vi "4.1 CSM API String to Numeric - Floating.vi"() -> ()   [LabVIEW 2017]
uses:
  63d4ee60-3d36-44f6-9846-d3c89712fa4e.vi
  5d5e870e-b8ec-4111-8fcd-715cbb1e366c.vi
  6ca2ea0b-5a64-4cad-9736-18ec21bbeae0.vi
  4ee676fc-47c0-4be0-9ff8-88677d132e6f.vi
  a152669e-7808-472e-ac68-82058263c032.vi
  API-String-Arugments-Support/_Support/Data To API String Arguments.vi
  API-String-Arugments-Support/_Support/Convert API String Arguments to Data(variant).vi
panel:
  out "Array 3":T1(array[cluster])=[{"Inplut String (Arguments)"="1", "Data"=1.0, "error"={"status"=FALSE, "code"=0, "source"=""}}, {"Inplut String (Arguments)"="10", "Data"=10.0, "error"={"status"=FALSE, "code"=0, "source"=""}}, {"Inplut String (Arguments)"="100", "Data"=100.0, "error"={"status"=FALSE, "code"=0, "source"=""}}, {"Inplut String (Arguments)"="1000", "Data"=1000.0, "error"={"status"=FALSE, "code"=0, "source"=""}}, {"Inplut String (Arguments)"="10000", "Data"=10000.0, "error"={"status"=FALSE, "code"=0, "source"=""}}, {"Inplut String (Arguments)"="100000", "Data"=100000.0, "error"={"status"=FALSE, "code"=0, "source"=""}}, {"Inplut String (Arguments)"="1000000", "Data"=1000000.0, "error"={"status"=FALSE, "code"=0, "source"=""}}, {"Inplut String (Arguments)"="10000000", "Data"=10000000.0, "error"={"status"=FALSE, "code"=0, "source"=""}}, {"Inplut String (Arguments)"="100000000", "Data"=100000000.0, "error"={"status"=FALSE, "code"=0, "source"=""}}, {"Inplut String (Arguments)"="1000000000", "Data"=1000000000.0, "error"={"status"=FALSE, "code"=0, "source"=""}}, {"Inplut String (Arguments)"="10000000000", "Data"=10000000000.0, "error"={"status"=FALSE, "code"=0, "source"=""}}, {"Inplut String (Arguments)"="100000000000", "Data"=100000000000.0, "error"={"status"=FALSE, "code"=0, "source"=""}}, {"Inplut String (Arguments)"="1000000000000", "Data"=1000000000000.0, "error"={"status"=FALSE, "code"=0, "source"=""}}, {"Inplut String (Arguments)"="10000000000000", "Data"=10000000000000.0, "error"={"status"=FALSE, "code"=0, "source"=""}}, {"Inplut String (Arguments)"="100000000000000", "Data"=100000000000000.0, "error"={"status"=FALSE, "code"=0, "source"=""}}, {"Inplut String (Arguments)"="1000000000000000", "Data"=1000000000000000.0, "error"={"status"=FALSE, "code"=0, "source"=""}}, {"Inplut String (Arguments)"="10000000000000000", "Data"=1e+16, "error"={"status"=FALSE, "code"=0, "source"=""}}, {"Inplut String (Arguments)"="100000000000000000", "Data"=1e+17, "error"={"status"=FALSE, "code"=0, "source"=""}}, {"Inplut String (Arguments)"="1000000000000000000", "Data"=1e+18, "error"={"status"=FALSE, "code"=0, "source"=""}}, {"Inplut String (Arguments)"="10000000000000000000", "Data"=1e+19, "error"={"status"=FALSE, "code"=0, "source"=""}}, {"Inplut String (Arguments)"="100000000000000000000", "Data"=1e+20, "error"={"status"=FALSE, "code"=0, "source"=""}}, {"Inplut String (Arguments)"="1000000000000000000000", "Data"=1e+21, "error"={"status"=FALSE, "code"=0, "source"=""}}, {"Inplut String (Arguments)"="10000000000000000000000", "Data"=1e+22, "error"={"status"=FALSE, "code"=0, "source"=""}}, {"Inplut String (Arguments)"="100000000000000000000000", "Data"=1e+23, "error"={"status"=FALSE, "code"=0, "source"=""}}, {"Inplut String (Arguments)"="1000000000000000000000000", "Data"=1e+24, "error"={"status"=FALSE, "code"=0, "source"=""}}, {"Inplut String (Arguments)"="10000000000000000000000000", "Data"=1e+25, "error"={"status"=FALSE, "code"=0, "source"=""}}, {"Inplut String (Arguments)"="100000000000000000000000000", "Data"=1e+26, "error"={"status"=FALSE, "code"=0, "source"=""}}, {"Inplut String (Arguments)"="1000000000000000000000000000", "Data"=1e+27, "error"={"status"=FALSE, "code"=0, "source"=""}}, {"Inplut String (Arguments)"="10000000000000000000000000000", "Data"=1e+28, "error"={"status"=FALSE, "code"=0, "source"=""}}, {"Inplut String (Arguments)"="100000000000000000000000000000", "Data"=1e+29, "error"={"status"=FALSE, "code"=0, "source"=""}}, {"Inplut String (Arguments)"="1000000000000000000000000000000", "Data"=1e+30, "error"={"status"=FALSE, "code"=0, "source"=""}}, {"Inplut String (Arguments)"="10000000000000000000000000000000", "Data"=1e+31, "error"={"status"=FALSE, "code"=0, "source"=""}}, {"Inplut String (Arguments)"="100000000000000000000000000000000", "Data"=1e+32, "error"={"status"=FALSE, "code"=0, "source"=""}}, {"Inplut String (Arguments)"="1000000000000000000000000000000000", "Data"=1e+33, "error"={"status"=FALSE, "code"=0, "source"=""}}, {"Inplut String (Arguments)"="10000000000000000000000000000000000", "Data"=1e+34, "error"={"status"=FALSE, "code"=0, "source"=""}}] {"Data" format="%#_6e"}
  out "Multiplication Display":T2(array[cluster])=[{"Float Value"=10.001, "Flatten String"="10.001", "Retrieve Float"=10.001, "error"={"status"=FALSE, "code"=0, "source"=""}}, {"Float Value"=100.00999999999999, "Flatten String"="100.01", "Retrieve Float"=100.01, "error"={"status"=FALSE, "code"=0, "source"=""}}, {"Float Value"=1000.0999999999999, "Flatten String"="1.0001k", "Retrieve Float"=1000.1, "error"={"status"=FALSE, "code"=0, "source"=""}}, {"Float Value"=10001.0, "Flatten String"="10.001k", "Retrieve Float"=10001.0, "error"={"status"=FALSE, "code"=0, "source"=""}}, {"Float Value"=100010.0, "Flatten String"="100.01k", "Retrieve Float"=100010.0, "error"={"status"=FALSE, "code"=0, "source"=""}}, {"Float Value"=1000100.0, "Flatten String"="1.0001M", "Retrieve Float"=1000100.0, "error"={"status"=FALSE, "code"=0, "source"=""}}, {"Float Value"=10001000.0, "Flatten String"="10.001M", "Retrieve Float"=10001000.0, "error"={"status"=FALSE, "code"=0, "source"=""}}, {"Float Value"=100010000.0, "Flatten String"="100.01M", "Retrieve Float"=100010000.0, "error"={"status"=FALSE, "code"=0, "source"=""}}, {"Float Value"=1000100000.0, "Flatten String"="1.0001G", "Retrieve Float"=1000100000.0, "error"={"status"=FALSE, "code"=0, "source"=""}}, {"Float Value"=10001000000.0, "Flatten String"="10.001G", "Retrieve Float"=10001000000.0, "error"={"status"=FALSE, "code"=0, "source"=""}}, {"Float Value"=100010000000.0, "Flatten String"="100.01G", "Retrieve Float"=100010000000.0, "error"={"status"=FALSE, "code"=0, "source"=""}}, {"Float Value"=1000100000000.0, "Flatten String"="1.0001T", "Retrieve Float"=1000100000000.0, "error"={"status"=FALSE, "code"=0, "source"=""}}, {"Float Value"=10001000000000.0, "Flatten String"="10.001T", "Retrieve Float"=10001000000000.0, "error"={"status"=FALSE, "code"=0, "source"=""}}, {"Float Value"=100010000000000.0, "Flatten String"="100.01T", "Retrieve Float"=100010000000000.0, "error"={"status"=FALSE, "code"=0, "source"=""}}, {"Float Value"=1000100000000000.0, "Flatten String"="1.0001P", "Retrieve Float"=1000100000000000.0, "error"={"status"=FALSE, "code"=0, "source"=""}}, {"Float Value"=1.0001e+16, "Flatten String"="10.001P", "Retrieve Float"=1.0001e+16, "error"={"status"=FALSE, "code"=0, "source"=""}}, {"Float Value"=1.0001e+17, "Flatten String"="100.01P", "Retrieve Float"=1.0001e+17, "error"={"status"=FALSE, "code"=0, "source"=""}}, {"Float Value"=1.0001e+18, "Flatten String"="1.0001E", "Retrieve Float"=1.0001e+18, "error"={"status"=FALSE, "code"=0, "source"=""}}, {"Float Value"=1.0001e+19, "Flatten String"="10.001E", "Retrieve Float"=1.0001e+19, "error"={"status"=FALSE, "code"=0, "source"=""}}, {"Float Value"=1.0001e+20, "Flatten String"="100.01E", "Retrieve Float"=1.0001e+20, "error"={"status"=FALSE, "code"=0, "source"=""}}, {"Float Value"=1.0001e+21, "Flatten String"="1.0001Z", "Retrieve Float"=1.0001e+21, "error"={"status"=FALSE, "code"=0, "source"=""}}, {"Float Value"=1.0001e+22, "Flatten String"="10.001Z", "Retrieve Float"=1.0001e+22, "error"={"status"=FALSE, "code"=0, "source"=""}}, {"Float Value"=1.0001e+23, "Flatten String"="100.01Z", "Retrieve Float"=1.0001000000000001e+23, "error"={"status"=FALSE, "code"=0, "source"=""}}, {"Float Value"=1.0000999999999999e+24, "Flatten String"="1.0001Y", "Retrieve Float"=1.0000999999999999e+24, "error"={"status"=FALSE, "code"=0, "source"=""}}, {"Float Value"=1.0001e+25, "Flatten String"="10.001Y", "Retrieve Float"=1.0001e+25, "error"={"status"=FALSE, "code"=0, "source"=""}}, {"Float Value"=1.0001e+26, "Flatten String"="100.01Y", "Retrieve Float"=1.0001000000000001e+26, "error"={"status"=FALSE, "code"=0, "source"=""}}, {"Float Value"=1.0001e+27, "Flatten String"="1.000100E+27", "Retrieve Float"=1.0001e+27, "error"={"status"=FALSE, "code"=0, "source"=""}}, {"Float Value"=1.0001e+28, "Flatten String"="10.001000E+27", "Retrieve Float"=1.0000999999999999e+28, "error"={"status"=FALSE, "code"=0, "source"=""}}, {"Float Value"=1.0001e+29, "Flatten String"="100.010000E+27", "Retrieve Float"=1.0001e+29, "error"={"status"=FALSE, "code"=0, "source"=""}}, {"Float Value"=1.0001e+30, "Flatten String"="1.000100E+30", "Retrieve Float"=1.0001e+30, "error"={"status"=FALSE, "code"=0, "source"=""}}, {"Float Value"=1.0001e+31, "Flatten String"="10.001000E+30", "Retrieve Float"=1.0001e+31, "error"={"status"=FALSE, "code"=0, "source"=""}}, {"Float Value"=1.0001e+32, "Flatten String"="100.010000E+30", "Retrieve Float"=1.0001000000000001e+32, "error"={"status"=FALSE, "code"=0, "source"=""}}, {"Float Value"=1.0001e+33, "Flatten String"="1.000100E+33", "Retrieve Float"=1.0001e+33, "error"={"status"=FALSE, "code"=0, "source"=""}}, {"Float Value"=1.0001e+34, "Flatten String"="10.001000E+33", "Retrieve Float"=1.0000999999999999e+34, "error"={"status"=FALSE, "code"=0, "source"=""}}, {"Float Value"=1.0001e+35, "Flatten String"="100.010000E+33", "Retrieve Float"=1.0001e+35, "error"={"status"=FALSE, "code"=0, "source"=""}}] {"Float Value" format="%#_6e"; "Retrieve Float" format="%#_6e"}
  out "Division Demonstration":T2(array[cluster])=[{"Float Value"=0.10001, "Flatten String"="100.01m", "Retrieve Float"=0.10001, "error"={"status"=FALSE, "code"=0, "source"=""}}, {"Float Value"=0.010001, "Flatten String"="10.001m", "Retrieve Float"=0.010001, "error"={"status"=FALSE, "code"=0, "source"=""}}, {"Float Value"=0.0010000999999999999, "Flatten String"="1.0001m", "Retrieve Float"=0.0010001, "error"={"status"=FALSE, "code"=0, "source"=""}}, {"Float Value"=0.00010000999999999999, "Flatten String"="100.01u", "Retrieve Float"=0.00010001, "error"={"status"=FALSE, "code"=0, "source"=""}}, {"Float Value"=1.0000999999999998e-05, "Flatten String"="10.001u", "Retrieve Float"=1.0001e-05, "error"={"status"=FALSE, "code"=0, "source"=""}}, {"Float Value"=1.0000999999999998e-06, "Flatten String"="1.0001u", "Retrieve Float"=1.0001e-06, "error"={"status"=FALSE, "code"=0, "source"=""}}, {"Float Value"=1.0000999999999998e-07, "Flatten String"="100.01n", "Retrieve Float"=1.0001000000000001e-07, "error"={"status"=FALSE, "code"=0, "source"=""}}, {"Float Value"=1.0000999999999998e-08, "Flatten String"="10.001n", "Retrieve Float"=1.0001e-08, "error"={"status"=FALSE, "code"=0, "source"=""}}, {"Float Value"=1.0000999999999999e-09, "Flatten String"="1.0001n", "Retrieve Float"=1.0001e-09, "error"={"status"=FALSE, "code"=0, "source"=""}}, {"Float Value"=1.0000999999999999e-10, "Flatten String"="100.01p", "Retrieve Float"=1.0001e-10, "error"={"status"=FALSE, "code"=0, "source"=""}}, {"Float Value"=1.0000999999999998e-11, "Flatten String"="10.001p", "Retrieve Float"=1.0001e-11, "error"={"status"=FALSE, "code"=0, "source"=""}}, {"Float Value"=1.0000999999999997e-12, "Flatten String"="1.0001p", "Retrieve Float"=1.0001e-12, "error"={"status"=FALSE, "code"=0, "source"=""}}, {"Float Value"=1.0000999999999997e-13, "Flatten String"="100.01f", "Retrieve Float"=1.0001000000000001e-13, "error"={"status"=FALSE, "code"=0, "source"=""}}, {"Float Value"=1.0000999999999997e-14, "Flatten String"="10.001f", "Retrieve Float"=1.0001e-14, "error"={"status"=FALSE, "code"=0, "source"=""}}, {"Float Value"=1.0000999999999996e-15, "Flatten String"="1.0001f", "Retrieve Float"=1.0001e-15, "error"={"status"=FALSE, "code"=0, "source"=""}}, {"Float Value"=1.0000999999999996e-16, "Flatten String"="100.01a", "Retrieve Float"=1.0001000000000001e-16, "error"={"status"=FALSE, "code"=0, "source"=""}}, {"Float Value"=1.0000999999999996e-17, "Flatten String"="10.001a", "Retrieve Float"=1.0001e-17, "error"={"status"=FALSE, "code"=0, "source"=""}}, {"Float Value"=1.0000999999999996e-18, "Flatten String"="1.0001a", "Retrieve Float"=1.0001e-18, "error"={"status"=FALSE, "code"=0, "source"=""}}, {"Float Value"=1.0000999999999995e-19, "Flatten String"="100.01z", "Retrieve Float"=1.0000999999999999e-19, "error"={"status"=FALSE, "code"=0, "source"=""}}, {"Float Value"=1.0000999999999996e-20, "Flatten String"="10.001z", "Retrieve Float"=1.0000999999999999e-20, "error"={"status"=FALSE, "code"=0, "source"=""}}, {"Float Value"=1.0000999999999995e-21, "Flatten String"="1.0001z", "Retrieve Float"=1.0001e-21, "error"={"status"=FALSE, "code"=0, "source"=""}}, {"Float Value"=1.0000999999999995e-22, "Flatten String"="100.01y", "Retrieve Float"=1.0001e-22, "error"={"status"=FALSE, "code"=0, "source"=""}}, {"Float Value"=1.0000999999999995e-23, "Flatten String"="10.001y", "Retrieve Float"=1.0000999999999998e-23, "error"={"status"=FALSE, "code"=0, "source"=""}}, {"Float Value"=1.0000999999999995e-24, "Flatten String"="1.0001y", "Retrieve Float"=1.0000999999999998e-24, "error"={"status"=FALSE, "code"=0, "source"=""}}, {"Float Value"=1.0000999999999995e-25, "Flatten String"="100.010000E-27", "Retrieve Float"=1.0001000000000001e-25, "error"={"status"=FALSE, "code"=0, "source"=""}}, {"Float Value"=1.0000999999999995e-26, "Flatten String"="10.001000E-27", "Retrieve Float"=1.0001e-26, "error"={"status"=FALSE, "code"=0, "source"=""}}, {"Float Value"=1.0000999999999995e-27, "Flatten String"="1.000100E-27", "Retrieve Float"=1.0001e-27, "error"={"status"=FALSE, "code"=0, "source"=""}}, {"Float Value"=1.0000999999999995e-28, "Flatten String"="100.010000E-30", "Retrieve Float"=1.0001000000000002e-28, "error"={"status"=FALSE, "code"=0, "source"=""}}, {"Float Value"=1.0000999999999995e-29, "Flatten String"="10.001000E-30", "Retrieve Float"=1.0001000000000001e-29, "error"={"status"=FALSE, "code"=0, "source"=""}}, {"Float Value"=1.0000999999999995e-30, "Flatten String"="1.000100E-30", "Retrieve Float"=1.0001e-30, "error"={"status"=FALSE, "code"=0, "source"=""}}, {"Float Value"=1.0000999999999994e-31, "Flatten String"="100.010000E-33", "Retrieve Float"=1.0001e-31, "error"={"status"=FALSE, "code"=0, "source"=""}}, {"Float Value"=1.0000999999999994e-32, "Flatten String"="10.001000E-33", "Retrieve Float"=1.0001e-32, "error"={"status"=FALSE, "code"=0, "source"=""}}, {"Float Value"=1.0000999999999995e-33, "Flatten String"="1.000100E-33", "Retrieve Float"=1.0001e-33, "error"={"status"=FALSE, "code"=0, "source"=""}}, {"Float Value"=1.0000999999999995e-34, "Flatten String"="100.010000E-36", "Retrieve Float"=1.0001e-34, "error"={"status"=FALSE, "code"=0, "source"=""}}, {"Float Value"=1.0000999999999996e-35, "Flatten String"="10.001000E-36", "Retrieve Float"=1.0001e-35, "error"={"status"=FALSE, "code"=0, "source"=""}}] {"Float Value" format="%#_6e"; "Retrieve Float" format="%#_6e"}
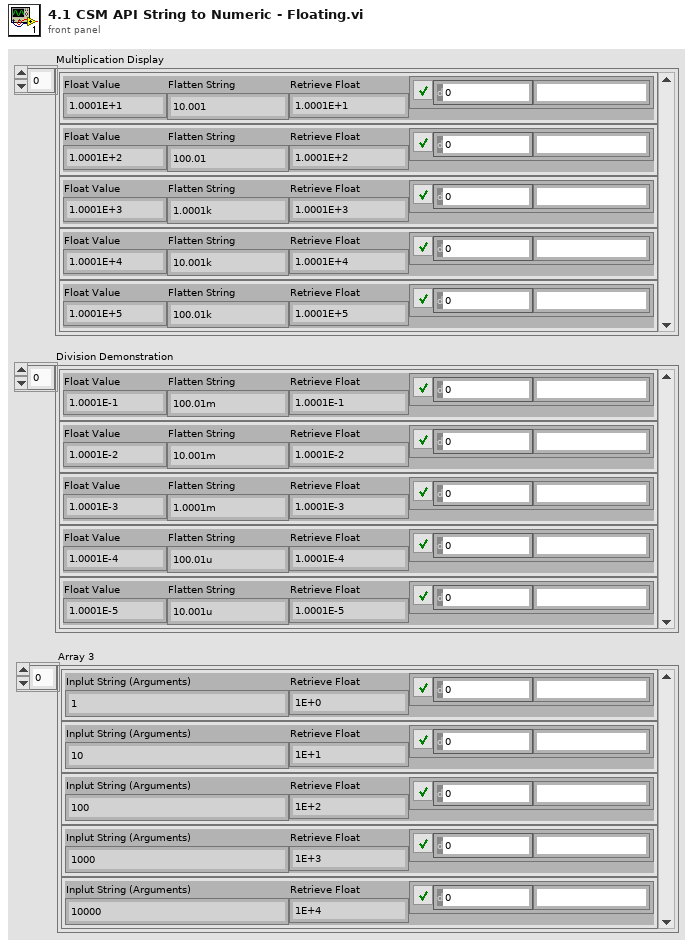
[diagram p1: front panel]
types:
  T1 = cluster{"Inplut String (Arguments)":string, "Data":dbl, "error":errorcluster}[]
  T2 = cluster{"Float Value":dbl, "Flatten String":string, "Retrieve Float":dbl, "error":errorcluster}[]
  T3 = cluster{dbl, "String":string, "Data":dbl, "error":errorcluster}
  T4 = cluster{"string":string, "Data":dbl, "error":errorcluster}
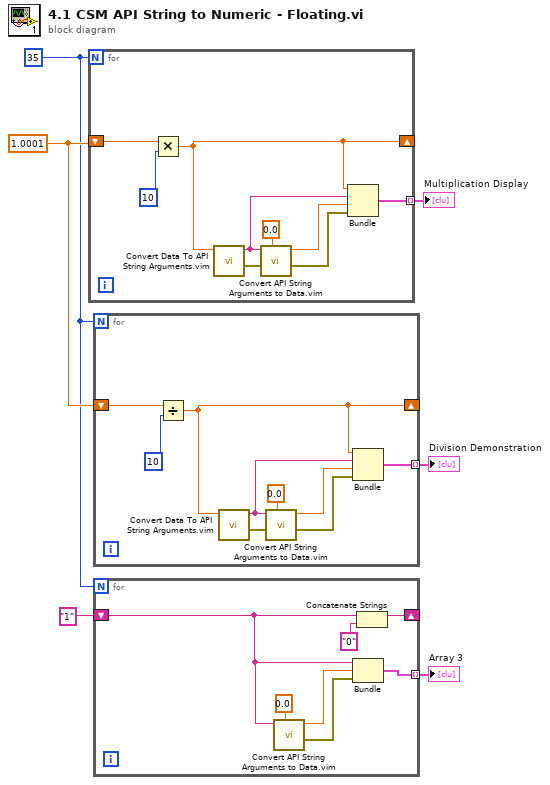
[diagram p0: block diagram]
diagram:
  w4 = 1.0001
  w2 = 35
  n1 = for {
    N: w2 -> [_]
    shift-right: [w11] -> _
    shift-left: w4 -> [w14]
    tunnel: [w7] -> w5 mode=indexing
    n2 = Multiply(x=w14, y=10) -> (x*y=w11:dbl)
    n3 = call "Convert Data To API String Arguments.vim"("data"=w11) -> ("error out"=w12:errorcluster, "String"=w10:string)  [unwired: 7 in]
    n4 = call "Convert API String Arguments to Data.vim"("Type"=0.0, "error in (no error)"=w12, "String"=w10) -> ("error"=w8:errorcluster, "Data"=w9:dbl)  [unwired: 5 in]
    n5 = Bundle(w11, "String"=w10, "Data"=w9, "error"=w8) -> (w7:T3)  [unwired: 1 in]
  }
  "Multiplication Display" <- w5
  n6 = for {
    N: w2 -> [_]
    shift-right: [w20] -> _
    shift-left: w4 -> [w23]
    tunnel: [w16] -> w6 mode=indexing
    n7 = Divide(x=w23, y=10) -> (x/y=w20:dbl)
    n8 = call "Convert Data To API String Arguments.vim"("data"=w20) -> ("error out"=w21:errorcluster, "String"=w19:string)  [unwired: 7 in]
    n9 = call "Convert API String Arguments to Data.vim"("Type"=0.0, "error in (no error)"=w21, "String"=w19) -> ("error"=w17:errorcluster, "Data"=w18:dbl)  [unwired: 5 in]
    n10 = Bundle(w20, "String"=w19, "Data"=w18, "error"=w17) -> (w16:T3)  [unwired: 1 in]
  }
  "Division Demonstration" <- w6
  n11 = for {
    N: w2 -> [_]
    shift-right: [w27] -> _
    shift-left: "1" ("string") -> [w25]
    tunnel: [w28] -> w3 mode=indexing
    n12 = call "Convert API String Arguments to Data.vim"("Type"=0.0, "String"=w25) -> ("error"=w29:errorcluster, "Data"=w30:dbl)  [unwired: 6 in]
    n13 = Bundle("string"=w25, "Data"=w30, "error"=w29) -> (w28:T4)  [unwired: 1 in]
    n14 = Concatenate Strings(w25, "0" ("string")) -> (w27:string)
  }
  "Array 3" <- w3
